vi "read sequencer status update.vi"(8 "error in (no error)":errorcluster, 9 "timeout (1 ms)":i32=1, 10 "output action status?":bool, 11 "Simple Sequencer API in":refnum<class "Simple Sequencer API.lvclass">) -> (0 "error out":errorcluster, 1 "Sequencer Stopped":bool, 2 "Status String":string, 3 "Simple Sequencer API out":refnum<class "Simple Sequencer API.lvclass">, 4 "Sequence Complete":bool)   [LabVIEW 2015, in "Simple Sequencer API.lvclass"]
doc: "Returns state information from the sequencer.\n\noutput action status? - determines whether or not this VI returns information when each action completes in addition to the general status information of the sequencer.\n\ntimeout - specifies how long to block waiting for a new status update."
uses:
  Simple Sequencer API.lvclass
  Simple Sequencer API.lvclass/Simple Sequencer API.ctl
  module/execution/sequencer states.ctl
  <vilib>/NI/AMC/Read Termination Message.vi
  <vilib>/NI/AMC/Create Single Message.vi
  <vilib>/NI/AMC/Globals.vi
  sequencer parent classes/action configuration parent/action configuration.lvclass
  <vilib>/NI/AMC/AMC.lvlib
  module/execution/Simple Sequencer TBM runtime.lvclass
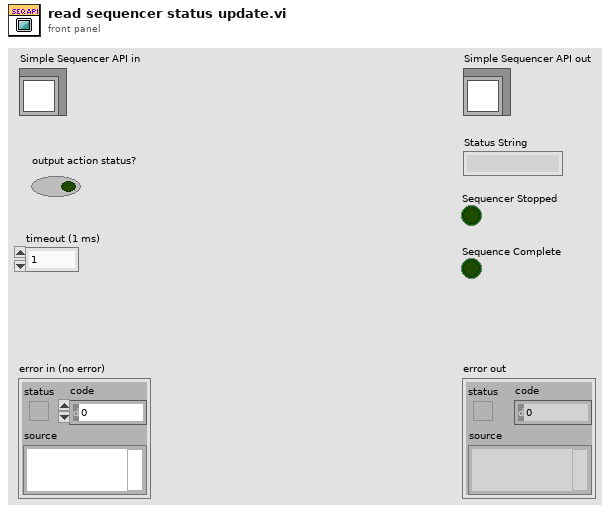
[diagram p1: front panel]
types:
  T1 = typedef "Simple Sequencer TBM runtime.lvclass/sequencer states.ctl" = enum16{"stopped", "running", "paused"}
  T2 = typedef "AMC.lvlib/Message Queue.ctl" = refnum<queue>
  T3 = typedef "Simple Sequencer TBM configuration.lvclass/sequence definition.ctl" = cluster{"sequence name":string, "action configs":refnum<class "action configuration.lvclass">[]}
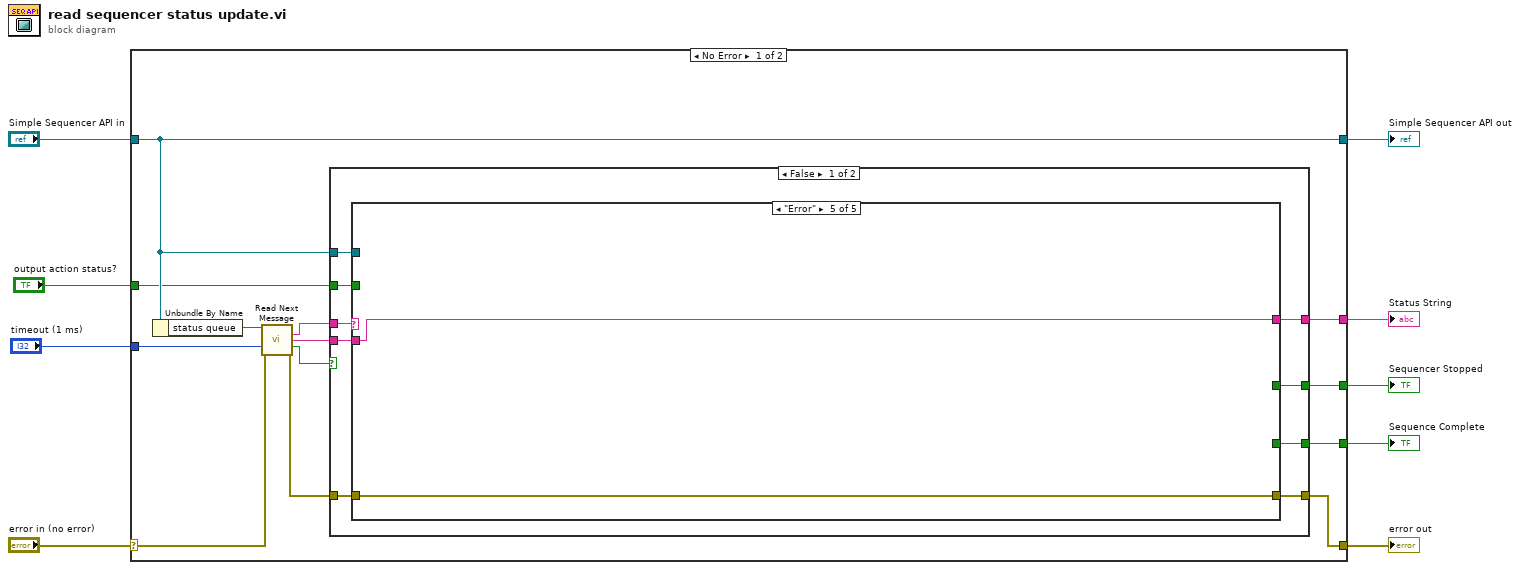
[diagram p0: block diagram]
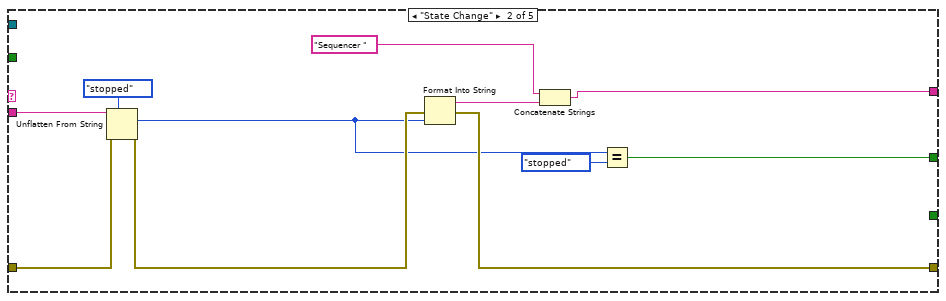
[diagram p3: hidden frame]
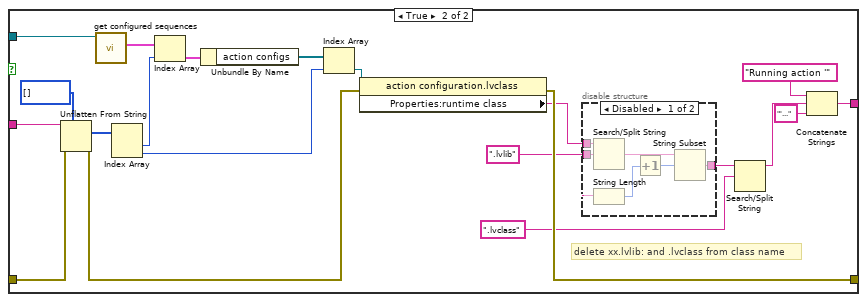
[diagram p5: hidden frame]
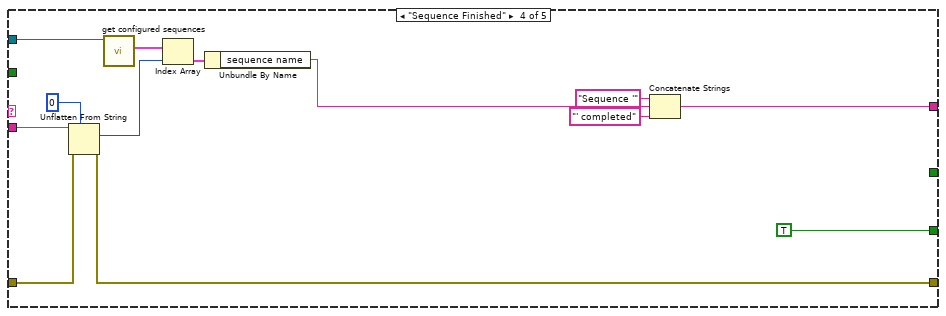
[diagram p7: hidden frame]
diagram:
  n1 = case shown="No Error" "error in (no error)" {
    selector: "error in (no error)" -> [w20 w96]
    tunnel: [w15 w96] -> w8
    tunnel: [w14 w95] -> w6
    tunnel: "Simple Sequencer API in" -> [w14 w95]
    tunnel: "timeout (1 ms)" -> [w21 _]
    tunnel: [w13 _] -> w4
    tunnel: [w12 _] -> w3
    tunnel: "output action status?" -> [w11 _]
    tunnel: [w10 _] -> w1
    frame No Error {
      n2 = Unbundle By Name(w14) -> ("status queue"=w22:T2)
      n3 = call <vilib>:"Read Next Message.vi"("message queue in"=w22, "timeout (1 ms)"=w21, "error in"=w20) -> ("message name"=w18:string, "message value"=w17:string, "timed out?"=w19:bool, "error out"=w16:errorcluster)  [unwired: 5 in, 4 out]
      n4 = case shown="False" w19 {
        tunnel: w18 -> [w31 _]
        tunnel: w17 -> [w30 _]
        tunnel: w16 -> [w29 w94]
        tunnel: [w28 w94] -> w15
        tunnel: w14 -> [w27 _]
        tunnel: [w26 _] -> w13
        tunnel: [w25 _] -> w12
        tunnel: w11 -> [w24 _]
        tunnel: [w23 _] -> w10
        frame False {
          n5 = case shown="\"Error\"" w31 {
            tunnel: w30 -> [_ w41 w49 w91 w93]
            tunnel: w29 -> [w32 w43 w48 w90 w92]
            tunnel: [w32 w39 w45 w89 w92] -> w28
            tunnel: w27 -> [_ _ w47 w88 _]
            tunnel: [_ w36 w46 w83 w93] -> w26
            tunnel: [_ w33 _ _ _] -> w25
            tunnel: w24 -> [_ _ w44 _ _]
            tunnel: [_ _ _ TRUE _] -> w23
            frame Default {
              # "#todo throw unrec msg error"
            }
            frame "State Change" {
              n6 = Unflatten From String(type=sequencer_states."stopped" ("state"), binary string=w41, error in (no error)=w43) -> (value=w35:T1, error out=w40:errorcluster)  [unwired: 2 in, 1 out]
              n7 = Format Into String(error in=w40, w35) -> (resulting string=w38:string, error out=w39:errorcluster)  [unwired: 2 in]
              n8 = Concatenate Strings("Sequencer ", w38) -> (w36:string)
              n9 = Equal?(x=w35, y=sequencer_states."stopped") -> (x = y?=w33:bool)
            }
            frame "Running Action" {
              n10 = case shown="False" w44 {
                tunnel: w49 -> [_ w71]
                tunnel: w48 -> [w50 w70]
                tunnel: w47 -> [_ w68]
                tunnel: [_ w58] -> w46
                tunnel: [w50 w56] -> w45
                frame False {
                }
                frame True {
                  # "delete xx.lvlib: and .lvclass from class name"
                  n11 = Unflatten From String(type=i32[] [] ("appended array"), binary string=w71, error in (no error)=w70) -> (value=w66:i32[], error out=w57:errorcluster)  [unwired: 2 in, 1 out]
                  n12 = call "get configured sequences.vi"("Simple Sequencer API in"=w68) -> ("sequence definitions"=w67:T3[])  [unwired: 8 in, 2 out]
                  n13 = Index Array(array=w66) -> (element #1=w65:i32, element #2=w62:i32)  [unwired: 2 in]
                  n14 = Index Array(array=w67, index=w65) -> (element=w64:T3)
                  n15 = Unbundle By Name(w64) -> ("action configs"=w63:refnum<class "action configuration.lvclass">[])
                  n16 = Index Array(array=w63, index=w62) -> (element=w61:refnum<class "action configuration.lvclass">)
                  n17 = property class="action configuration.lvclass"(reference=w61, error in=w57) -> (error out=w56:errorcluster, "Properties:runtime class"=w55:string)  [unwired: 1 out]
                  n18 = disable-structure shown="Disabled" {
                    disable-tunnel: w55 -> [w77 w78]
                    disable-tunnel: ".lvlib" ("search string/char (-)") -> [w76 _]
                    disable-tunnel: [w74 w78] -> w53
                    frame Disabled {
                      n19 = Search/Split String(string=w77, search string/char (-)=w76) -> (match + rest of string=w75:string)  [unwired: 1 in, 2 out]
                      n20 = String Length(string=w76) -> (length=w73:i32)
                      n21 = Increment(x=w73) -> (x+1=w72:i32)
                      n22 = String Subset(string=w75, offset (0)=w72) -> (substring=w74:string)  [unwired: 1 in]
                    }
                    frame Enabled {
                    }
                  }
                  n23 = Search/Split String(string=w53, search string/char (-)=".lvclass") -> (substring before match=w51:string)  [unwired: 1 in, 2 out]
                  n24 = Concatenate Strings("Running action '" ("string"), w51, "'..." ("string")) -> (w58:string)
                }
              }
            }
            frame "Sequence Finished" {
              n25 = Unflatten From String(type=0 ("sequence index"), binary string=w91, error in (no error)=w90) -> (value=w81:i32, error out=w89:errorcluster)  [unwired: 2 in, 1 out]
              n26 = call "get configured sequences.vi"("Simple Sequencer API in"=w88) -> ("sequence definitions"=w87:T3[])  [unwired: 8 in, 2 out]
              n27 = Index Array(array=w87, index=w81) -> (element=w86:T3)
              n28 = Unbundle By Name(w86) -> ("sequence name"=w80:string)
              n29 = Concatenate Strings("Sequence '" ("string"), w80, "' completed" ("string")) -> (w83:string)
            }
            frame "Error" {
            }
          }
        }
        frame True {
        }
      }
    }
    frame Error {
    }
  }
  "error out" <- w8
  "Simple Sequencer API out" <- w6
  "Status String" <- w4
  "Sequencer Stopped" <- w3
  "Sequence Complete" <- w1
